vi "Diagnostics Request.vi"(8 "error in (no error)":errorcluster, 9 "Data":u16[](array[numeric]), 10 "Sub-function":T1 items=["Return Query Data"=0, "Restart Communications Option"=1, "Return Diagnostic Register"=2, "Change ASCII Input Delimiter"=3, "Force Listen Only Mode"=4, "Clear Counters and Diagnostic Register"=10, "Return Bus Message Count"=11, "Return Bus Communication Error Count"=12, "Return Bus Exception Error Count"=13, "Return Slave Message Count"=14, "Return Slave No Response Count"=15, "Return Slave NAK Count"=16, "Return Slave Busy Count"=17, "Return Bus Character Overrun Count"=18, "Clear Overrun Counter and Flag"=20]) -> (0 "error out":errorcluster, 2 "modbus data unit out":refnum<class "Modbus Data Unit.lvclass">)   [LabVIEW 2019, in "Modbus Library.lvlib" / "Master Function Definition.lvclass"]
uses:
  Master Function Definition.lvclass
  Diagnostics Subfuntion Options.ctl
  Modbus Data Unit/Modbus Data Unit.lvclass
  Modbus Data Unit/Function.ctl
  Modbus Data Unit/Modbus Data Unit.lvclass/Modbus Data Unit.ctl
  Modbus Library.lvlib
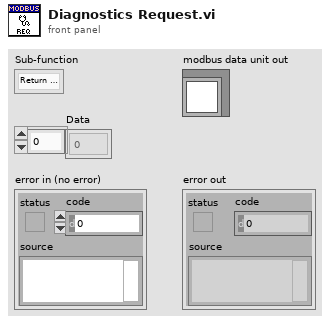
[diagram p1: front panel]
types:
  T1 = typedef "Modbus Library.lvlib/Master Function Definition.lvclass/Diagnostics Subfuntion Options.ctl" = u16
  T2 = typedef "Modbus Library.lvlib/Function.ctl" = u8
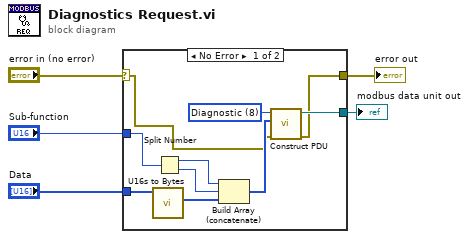
[diagram p0: block diagram]
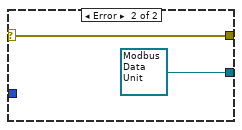
[diagram p2: hidden frame]
diagram:
  n1 = case shown="No Error" "error in (no error)" {
    selector: "error in (no error)" -> [w8 w17]
    tunnel: [w7 w17] -> w4
    tunnel: "Sub-function" -> [w13 _]
    tunnel: "Data" -> [w12 _]
    tunnel: [w9 refnum<class "Modbus Data Unit.lvclass"> refnum ("modbus data unit out")] -> w1
    frame No Error {
      w6 = T2 8 items=["Read Discrete Inputs"=2, "Read Coils"=1, "Write Single Coil"=5, "Write Multiple Coils"=15, "Read Input Register"=4, "Read Holding Registers"=3, "Write Single Register"=6, "Write Multiple Registers"=16, "Read/Write Multiple Registers"=23, "Mask Write Register"=22, "Read FIFO Queue"=24, "Read File Record"=20, "Write File Record"=21, "Read Exception Status"=7, "Diagnostic"=8, "Get Com Event Counter"=11, "Get Com Event Log"=12, "Report Slave ID"=17, "Read Device Identification"=43] ("Function")
      n2 = call "U16s to Bytes.vi"("Registers"=w12) -> ("Bytes"=w11:u8[])  [unwired: 9 in, 1 out]
      n3 = Split Number(x=w13) -> (hi(x)=w14:u8, lo(x)=w15:u8)
      n4 = Build Array (concatenate)(w14, w15, w11) -> (w10:u8[])
      n5 = call "Construct PDU.vi"("error in"=w8, "data"=w10, "Function"=w6) -> ("error out"=w7:errorcluster, "modbus data unit out"=w9:refnum<class "Modbus Data Unit.lvclass">)  [unwired: 7 in]
    }
    frame Error {
    }
  }
  "error out" <- w4
  "modbus data unit out" <- w1
